vi "Sys config window-Get set control values_retd.vi"(8 "error in (no error)":errorcluster, 11 "Function":T28) -> (0 "error out":errorcluster, 2 "output cluster":T1={"Triggers output setup"=[], "General trigger settings"={"Trigger 1 function"=enum."Encoder trigger", "Triggers loop clock (MHz)"=80.0}, "AOL Properties"={"AOD 1 thickness (mm)"=118.0, "AOD 2 thickness (mm)"=115.0, "AOD 3 thickness (mm)"=110.0, "AOD 4 thickness (mm)"=135.0, "AOD 5 thickness (mm)"=135.0, "AOD 6 thickness (mm)"=135.0, "AOD 1-2 separation (mm)"=15.0, "AOD 2-3 separation (mm)"=15.0, "AOD 3-4 separation (mm)"=15.0, "AOD 4-5 separation (mm)"=15.0, "AOD 5-6 separation (mm)"=15.0, "AOD 1 X Offset"=15.0, "AOD 2 X Offset"=1.0, "AOD 3 X Offset"=1.0, "AOD 4 X Offset"=1.0, "AOD 1 Y Offset"=1.0, "AOD 2 Y Offset"=1.0, "AOD 3 Y Offset"=1.0, "AOD 4 Y Offset"=1.0, "AOD 1 X Direction"=0.0, "AOD 2 X Direction"=0.0, "AOD 3 X Direction"=0.0, "AOD 4 X Direction"=0.0, "AOD 1 Y Direction"=1.0, "AOD 2 Y Direction"=20000.0, "AOD 3 Y Direction"=20000.0, "AOD 4 Y Direction"=0.0046, "AOD 1 Centre (mm)"=15.0, "AOD 2 Centre (mm)"=50.0, "AOD 3 Centre (mm)"=50.0, "AOD 4 Centre (mm)"=50.0, "Timing Offset AOD 1"=0.0, "Timing Offset AOD 2"=0.0, "Timing Offset AOD 3"=0.0, "Timing Offset AOD 4"=0.0, "AOD Optical offset 1"=0.0, "AOD Optical offset 2"=0.0, "AOL aperture (mm)"=15.0, "AOL centre wavelength (nm)"=1.0, "AOL centre frequency (MHz)"=1.0, "Diffraction mode"=1.0, "Crystal length (mm)"=0.0, "Acoustic velocity (m/s)"=1.0, "Pair deflection ratio"=1.0, "AOD fill time (us)"=1.0, "AOD Ord. Refractive index"=2.22, "AOD ExtraOrd. Refractive index"=2.22}, "Calibration settings"={"Pockels cal.Zoom"=0, "Pockels cal.Dwell time (µs)"=0.0}, "Hardware Configuration"={"Microscope ID"="003", "Microscope Type"="AOLM", "Revision Number"="1.0.0.0", "Advanced Imaging"=FALSE, "Max Allowed Trial Length"=60.0, "Initial Scan Resolution"=512.0, "Initial Acceptance Angle"=5.0, "Dev. PC"=FALSE, "Swap XY on stage"=FALSE, "No of AOD"=0, "MC Supported"=FALSE, "Axial MC"=FALSE, "Computer MAC address"="", "Externalise Triggers"=FALSE, "Trigger HW config"={"Available Device List"=0, "Device Address"=""}, "DAQmx Chan"={"Pockels AO"="", "Hard shutter AO"="", "PMT AOs"="", "Galvo AOs"="", "Power meter AI"=""}, "XY stage available"=FALSE, "XY Stage"={"COM port"="", "XY stage available"=FALSE, "Baudrate"=0, "Type"=""}, "Z stage available"=FALSE, "Z Stage config cluster"={"COM port"="COM7", "Baudrate"=0, "Type"=""}, "Encoder available"=FALSE, "Encoder"={"IP address"="224.0.1.103", "Port"=7000, "Wheel radius (cm)"=16.0, "Encoder Trigger"=""}, "VidRec available"=FALSE, "Cam VidRec"={"DO flag-Video record"="", "DO flag-Trial start"=""}, "Laser Power Control HW config"={"Laser Power Control"="", "Laser Power Modulation Control"=enum."NI"}, "Laser 1 available"=FALSE, "Laser 1 config cluster"={"COM port"="COM7", "Baud Rate"=0, "Type"=""}, "Prechirper 1 available"=FALSE, "Prechirper 1 config cluster"={"Type"="", "Baud Rate"=0, "COM port"="COM7"}, "Control system.FPGA available?"=FALSE, "Control Sys. HW config"={"Control system.FPGA Type"=enum."Virtex 5", "Control system.Network adapter name"="", "Control system.MAC address"="", "Control system.Ethernet Port"=0, "Control system.Ethernet Port Opened"=FALSE}, "DAQ FPGA HW Config"={"Target"="RIO0", "input card type"=enum."AC Card"}}, "System Config"={"Laser wavelength (nm)"=920.0, "DAQ FPGA System"={"Clock Freq (MHz) "=200.0, "Samples Wait after Trigger"=5080, "AOD fill"=4900, "StartupDelay"=0, "Slip Cycle (clock cycles)"=600000, "Add Cycle"=TRUE}, "Control system"={"AOD 1 Amplitude"=0, "AOD 2 Amplitude"=0, "AOD 3 Amplitude"=0, "AOD 4 Amplitude"=0, "AOD 5 Amplitude"=0, "AOD 6 Amplitude"=0, "T0 (ns)"=0.0, "Ta (ns)"=0.0, "Data Time Interval (ns)"=0.0, "Ctrl FPGA Clock (MHz)"=240.0}}, "Calibration config."={"Current Objective"="", "Objective Settings"=[], "PreChirper Values Preset ?"=FALSE, "PreChirper Settings"=[], "PreChirper Constants"={"a 1"=0, "b 1"=0, "c 1"=0, "a 2"=0, "b 2"=0, "c 2"=0, "lmin"=0, "lmax"=0}}} {"System Config"."Control system"."Ctrl FPGA Clock (MHz)" min=80.0 max=500.0 step=1.0; "System Config"."Control system"."Data Time Interval (ns)" min=0.0 max=2048.0 step=1.0; "System Config"."Control system"."Ta (ns)" min=0.0 max=2048.0 step=1.0; "System Config"."Control system"."T0 (ns)" min=0.0 max=2048.0 step=1.0; "System Config"."Control system"."AOD 6 Amplitude" min=0 max=2048 step=1; "System Config"."Control system"."AOD 5 Amplitude" min=0 max=2048 step=1; "System Config"."Control system"."AOD 4 Amplitude" min=0 max=2048 step=1; "System Config"."Control system"."AOD 3 Amplitude" min=0 max=2048 step=1; "System Config"."Control system"."AOD 2 Amplitude" min=0 max=2048 step=1; "System Config"."Control system"."AOD 1 Amplitude" min=0 max=2048 step=1; "System Config"."Laser wavelength (nm)" min=800.0 max=1080.0 step=1.0; "Hardware Configuration"."Encoder"."Wheel radius (cm)" format="%#_13g"; "General trigger settings"."Triggers loop clock (MHz)" format="%#_13g"; "Triggers output setup"."Pulse width (us)" min=10 max=5000 step=1 format="%.0fµs"})   [LabVIEW 2020]
uses:
  Typedefs/HW config states enum.ctl
  Globals/Sys Config window globals.vi
  Configuration code/Calibration/Globals/gl_Calibration globals.vi
  Configuration code/Typedefs/Pockels Calibration settings cluster.ctl
  Global Variables/General Globals.vi
  Peripherals Control/Triggers/Typedefs/Trigger setup element cluster.ctl
  Peripherals Control/Triggers/Typedefs/Triggers output setup.ctl
  Typedefs/Trigger 1 selector enum.ctl
  Peripherals Control/Triggers/Typedefs/General trigger settings cluster.ctl
  Typedefs/XY Stage config cluster.ctl
  Typedefs/Cam VidRec HW config setup cluster.ctl
  Typedefs/Control Sys HW config cluster.ctl
  <vilib>/userDefined/High Color/nirio_resource_hc.ctl
  Typedefs/FPGA input type AC-DC.ctl
  Typedefs/DAQmx physical channels cluster.ctl
  Typedefs/Encoder config cluster.ctl
  Typedefs/Z Stage config cluster.ctl
  Typedefs/Triggers HW config.ctl
  Typedefs/Laser 1 config cluster.ctl
  Typedefs/PreChirper 1 config cluster.ctl
  Typedefs/Laser Power Control HW config.ctl
  Typedefs/Hardware Configuration settings.ctl
  RIG-SPECIFIC FILES/FPGA Refs/FPGA Ref.ctl
  Typedefs/DAQ FPGA system config.ctl
  Typedefs/CTRL system config.ctl
  Typedefs/System Configuration.ctl
  Configuration code/Typedefs/Initial config.ctl
  Typedefs/PreChirper constants.ctl
  Typedefs/Prechirper Cal Config.ctl
  Typedefs/Objective Config.ctl
  Typedefs/Calibration config.ctl
  Typedefs/AOD Settings-distilled.ctl
  Typedefs/General Setup.ctl
  Typedefs/PMT Voltage Range.ctl
  Typedefs/DAQ FPGA HW config cluster.ctl
  Visualisation/Functional Imaging Viewer/Typedefs/Get-Set-Clear Control.ctl
  Typedefs/AOL Properties Cluster.ctl
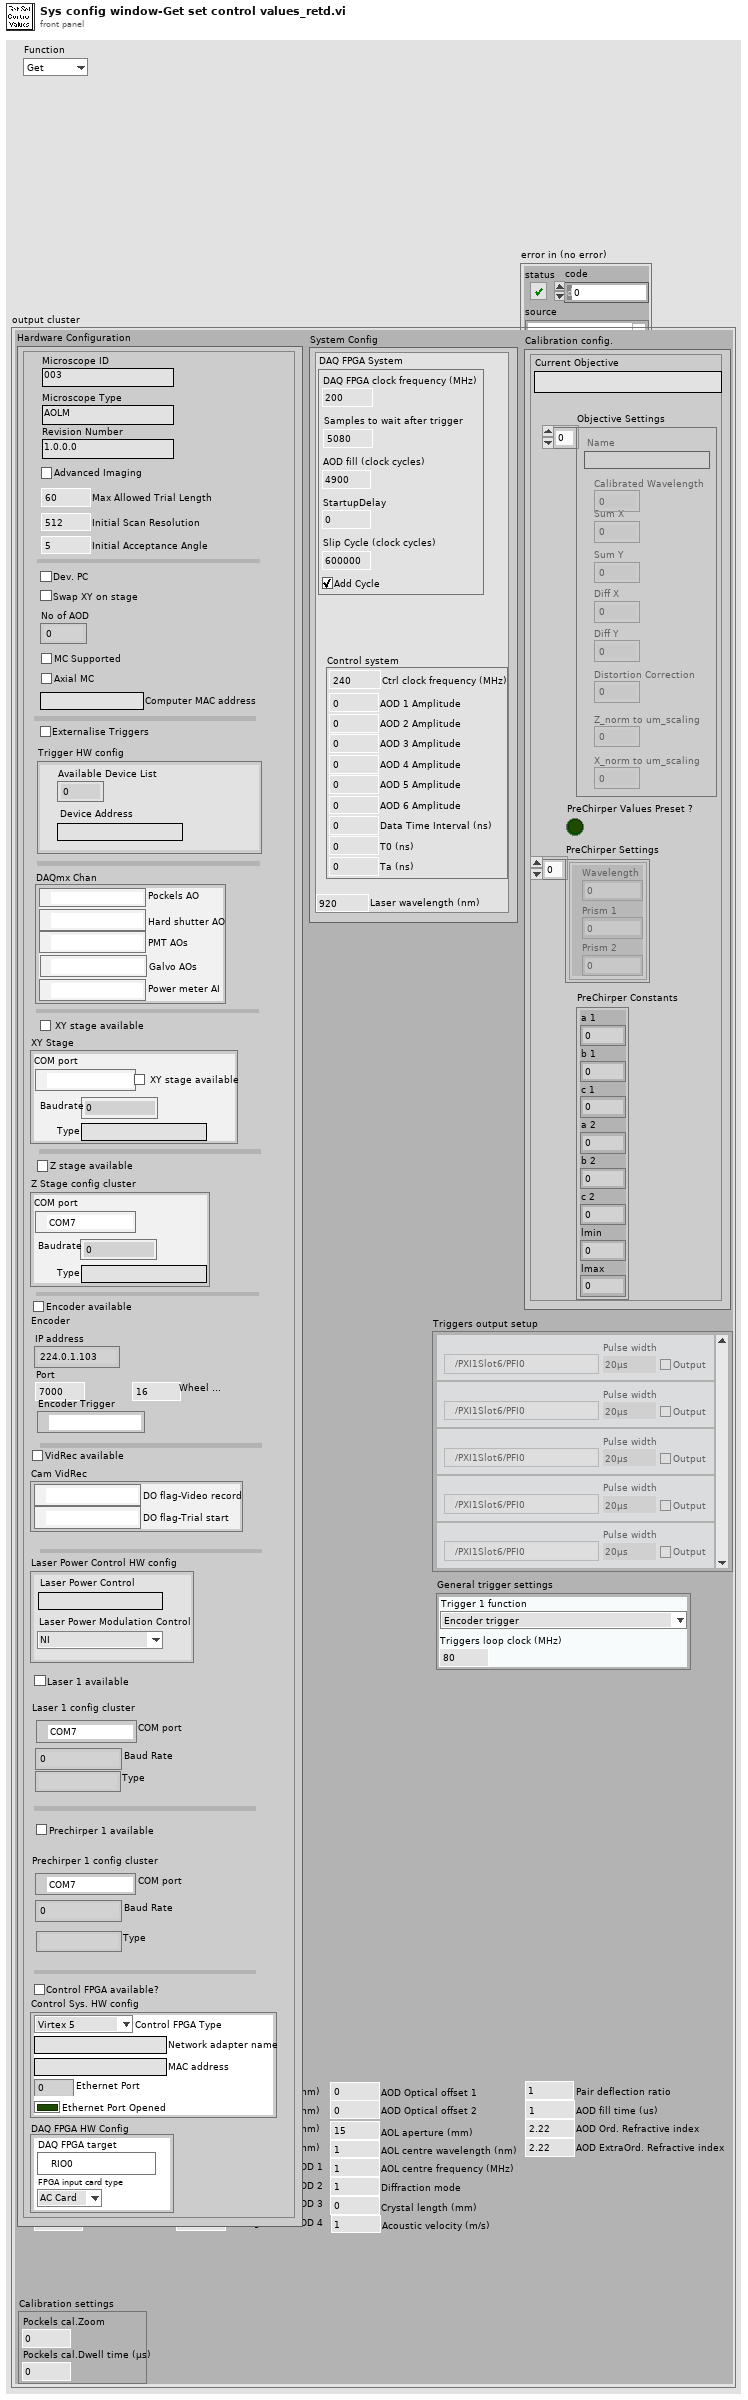
[diagram p1: front panel]
types:
  T1 = typedef "Initial config.ctl" = cluster{"Triggers output setup":T2, "General trigger settings":T4, "AOL Properties":T6, "Calibration settings":T7, "Hardware Configuration":T8, "System Config":T21, "Calibration config.":T24}
  T2 = typedef "Triggers output setup.ctl" = T3[]
  T3 = typedef "Trigger setup element cluster.ctl" = cluster{"Name":string, "Output?":bool, "Output terminal":tag, "PXI backplane line":tag, "Pulse width (us)":u16}
  T4 = typedef "General trigger settings cluster.ctl" = cluster{"Trigger 1 function":T5, "Triggers loop clock (MHz)":dbl}
  T5 = typedef "Trigger 1 selector enum.ctl" = enum16{"Encoder trigger", "Line trigger", "Control system's ref frame acknowledgement"}
  T6 = typedef "AOL Properties Cluster.ctl" = cluster{"AOD 1 thickness (mm)":dbl, "AOD 2 thickness (mm)":dbl, "AOD 3 thickness (mm)":dbl, "AOD 4 thickness (mm)":dbl, "AOD 5 thickness (mm)":dbl, "AOD 6 thickness (mm)":dbl, "AOD 1-2 separation (mm)":dbl, "AOD 2-3 separation (mm)":dbl, "AOD 3-4 separation (mm)":dbl, "AOD 4-5 separation (mm)":dbl, "AOD 5-6 separation (mm)":dbl, "AOD 1 X Offset":dbl, "AOD 2 X Offset":dbl, "AOD 3 X Offset":dbl, "AOD 4 X Offset":dbl, "AOD 1 Y Offset":dbl, "AOD 2 Y Offset":dbl, "AOD 3 Y Offset":dbl, "AOD 4 Y Offset":dbl, "AOD 1 X Direction":dbl, "AOD 2 X Direction":dbl, "AOD 3 X Direction":dbl, "AOD 4 X Direction":dbl, "AOD 1 Y Direction":dbl, "AOD 2 Y Direction":dbl, "AOD 3 Y Direction":dbl, "AOD 4 Y Direction":dbl, "AOD 1 Centre (mm)":dbl, "AOD 2 Centre (mm)":dbl, "AOD 3 Centre (mm)":dbl, "AOD 4 Centre (mm)":dbl, "Timing Offset AOD 1":dbl, "Timing Offset AOD 2":dbl, "Timing Offset AOD 3":dbl, "Timing Offset AOD 4":dbl, "AOD Optical offset 1":dbl, "AOD Optical offset 2":dbl, "AOL aperture (mm)":dbl, "AOL centre wavelength (nm)":dbl, "AOL centre frequency (MHz)":dbl, "Diffraction mode":dbl, "Crystal length (mm)":dbl, "Acoustic velocity (m/s)":dbl, "Pair deflection ratio":dbl, "AOD fill time (us)":dbl, "AOD Ord. Refractive index":dbl, "AOD ExtraOrd. Refractive index":dbl}
  T7 = typedef "Pockels Calibration settings cluster.ctl" = cluster{"Pockels cal.Zoom":u8, "Pockels cal.Dwell time (µs)":dbl}
  T8 = typedef "Hardware Configuration settings.ctl" = cluster{"Microscope ID":string, "Microscope Type":string, "Revision Number":string, "Advanced Imaging":bool, "Max Allowed Trial Length":dbl, "Initial Scan Resolution":dbl, "Initial Acceptance Angle":dbl, "Dev. PC":bool, "Swap XY on stage":bool, "No of AOD":u8, "MC Supported":bool, "Axial MC":bool, "Computer MAC address":string, "Externalise Triggers":bool, "Trigger HW config":T9, "DAQmx Chan":T10, "XY stage available":bool, "XY Stage":T11, "Z stage available":bool, "Z Stage config cluster":T12, "Encoder available":bool, "Encoder":T13, "VidRec available":bool, "Cam VidRec":T14, "Laser Power Control HW config":T15, "Laser 1 available":bool, "Laser 1 config cluster":T16, "Prechirper 1 available":bool, "Prechirper 1 config cluster":T17, "Control system.FPGA available?":bool, "Control Sys. HW config":T18, "DAQ FPGA HW Config":cluster{"Target":T19, "input card type":T20}}
  T9 = typedef "Triggers HW config.ctl" = cluster{"Available Device List":i32, "Device Address":string}
  T10 = typedef "DAQmx physical channels cluster.ctl" = cluster{"Pockels AO":tag, "Hard shutter AO":tag, "PMT AOs":tag, "Galvo AOs":tag, "Power meter AI":tag}
  T11 = typedef "XY Stage config cluster.ctl" = cluster{"COM port":refnum<visa-resource-name>, "XY stage available":bool, "Baudrate":i32, "Type":string}
  T12 = typedef "Z Stage config cluster.ctl" = cluster{"COM port":refnum<visa-resource-name>, "Baudrate":i32, "Type":string}
  T13 = typedef "Encoder config cluster.ctl" = cluster{"IP address":string, "Port":u16, "Wheel radius (cm)":dbl, "Encoder Trigger":tag}
  T14 = typedef "Cam VidRec HW config setup cluster.ctl" = cluster{"DO flag-Video record":tag, "DO flag-Trial start":tag}
  T15 = typedef "Laser Power Control HW config.ctl" = cluster{"Laser Power Control":string, "Laser Power Modulation Control":enum16{"NI", "FPGA"}}
  T16 = typedef "Laser 1 config cluster.ctl" = cluster{"COM port":refnum<visa-resource-name>, "Baud Rate":i32, "Type":string}
  T17 = typedef "PreChirper 1 config cluster.ctl" = cluster{"Type":string, "Baud Rate":i32, "COM port":refnum<visa-resource-name>}
  T18 = typedef "Control Sys HW config cluster.ctl" = cluster{"Control system.FPGA Type":enum16{"Virtex 5", "Virtex 7"}, "Control system.Network adapter name":string, "Control system.MAC address":string, "Control system.Ethernet Port":u32, "Control system.Ethernet Port Opened":bool}
  T19 = typedef "nirio_resource_hc.ctl" = tag
  T20 = typedef "FPGA input type AC-DC.ctl" = enum16{"AC Card", "DC Card"}
  T21 = typedef "System Configuration.ctl" = cluster{"Laser wavelength (nm)":dbl, "DAQ FPGA System":T22, "Control system":T23}
  T22 = typedef "DAQ FPGA system config.ctl" = cluster{"Clock Freq (MHz) ":dbl, "Samples Wait after Trigger":u16, "AOD fill":u16, "StartupDelay":i32, "Slip Cycle (clock cycles)":u32, "Add Cycle":bool}
  T23 = typedef "CTRL system config.ctl" = cluster{"AOD 1 Amplitude":i16, "AOD 2 Amplitude":i16, "AOD 3 Amplitude":i16, "AOD 4 Amplitude":i16, "AOD 5 Amplitude":i16, "AOD 6 Amplitude":i16, "T0 (ns)":dbl, "Ta (ns)":dbl, "Data Time Interval (ns)":dbl, "Ctrl FPGA Clock (MHz)":dbl}
  T24 = typedef "Calibration config.ctl" = cluster{"Current Objective":string, "Objective Settings":T25[], "PreChirper Values Preset ?":bool, "PreChirper Settings":T26[], "PreChirper Constants":T27}
  T25 = typedef "Objective Config.ctl" = cluster{"Name":string, "Sum X":dbl, "Sum Y":dbl, "Diff X":dbl, "Diff Y":dbl, "Distortion Correction":dbl, "Z_norm to um_scaling":dbl, "X_norm to um_scaling":dbl, "Calibrated Wavelength":dbl}
  T26 = typedef "Prechirper Cal Config.ctl" = cluster{"Wavelength":i32, "Prism 1":i32, "Prism 2":i32}
  T27 = typedef "PreChirper constants.ctl" = cluster{"a 1":i32, "b 1":i32, "c 1":i32, "a 2":i32, "b 2":i32, "c 2":i32, "lmin":i32, "lmax":i32}
  T28 = typedef "Get-Set-Clear Control.ctl" = enum16{"Get", "Set", "Clear"}
  T29 = enum16{"Initialise", "Load from file", "Save to file", "Read", "Write"}
  T30 = typedef "Initial config.ctl" = cluster{"Triggers output setup":T2, "General trigger settings":T4, "Calibration settings":T7, "Hardware Configuration":T31, "System Config":T21, "Calibration config.":T24, "General Setup":T36, "AOD Settings - distilled":T37}
  T31 = typedef "Hardware Configuration settings.ctl" = cluster{"Dev. PC":bool, "Swap XY on stage":bool, "No of AOD":u8, "MC Supported":bool, "Axial MC":bool, "Computer MAC address":string, "Externalise Triggers":bool, "Trigger HW config":T9, "DAQmx Chan":T10, "XY stage available":bool, "XY Stage":T32, "Z stage available":bool, "Z Stage config cluster":T12, "Encoder available":bool, "Encoder":T13, "VidRec available":bool, "Cam VidRec":T14, "Laser Power Control HW config":T15, "Laser 1 available":bool, "Laser 1 config cluster":T16, "Prechirper 1 available":bool, "Prechirper 1 config cluster":T17, "Control system.FPGA available?":bool, "Control Sys. HW config":T18, "DAQ FPGA HW Config":T33, "PMT Voltage Range":T35}
  T32 = typedef "XY Stage config cluster.ctl" = cluster{"COM port":refnum<visa-resource-name>, "Baudrate":i32, "Type":string}
  T33 = typedef "DAQ FPGA HW config cluster.ctl" = cluster{"FGPA Ref":T34, "Target":T19, "input card type":T20}
  T34 = typedef "FPGA Ref.ctl" = refnum<k20>
  T35 = typedef "PMT Voltage Range.ctl" = cluster{"PMT Voltage Lower Limit":dbl, "PMT Voltage Upper Limit":dbl}
  T36 = typedef "General Setup.ctl" = cluster{"Microscope ID":string, "Microscope Type":string, "Revision Number":string, "Advanced Imaging":bool, "Error Logging":bool, "Performance Monitoring":bool, "Max Allowed Trial Length":dbl, "Initial Scan Resolution":dbl, "Initial Acceptance Angle":dbl, "Initial Laser Wavelength":dbl, "Initial Dwell Time":dbl}
  T37 = typedef "AOD Settings-distilled.ctl" = cluster{"AOD 1 thickness (mm)":dbl, "AOD 2 thickness (mm)":dbl, "AOD 3 thickness (mm)":dbl, "AOD 4 thickness (mm)":dbl, "AOD 1-2 separation (mm)":dbl, "AOD 2-3 separation (mm)":dbl, "AOD 3-4 separation (mm)":dbl, "AOD 1 Centre (mm)":dbl, "AOD 2 Centre (mm)":dbl, "AOD 3 Centre (mm)":dbl, "AOD 4 Centre (mm)":dbl, "AOD 1 X Offset":dbl, "AOD 2 X Offset":dbl, "AOD 3 X Offset":dbl, "AOD 4 X Offset":dbl, "AOD 1 Y Offset":dbl, "AOD 2 Y Offset":dbl, "AOD 3 Y Offset":dbl, "AOD 4 Y Offset":dbl, "Timing Offset AOD 1":dbl, "Timing Offset AOD 2":dbl, "Timing Offset AOD 3":dbl, "Timing Offset AOD 4":dbl, "AOL centre wavelength (nm)":dbl, "AOL centre frequency (MHz)":dbl, "Pair deflection ratio":dbl, "AOL aperture (mm)":dbl, "AOD fill time (us)":dbl, "Diffraction mode":dbl, "Crystal length (mm)":dbl, "Acoustic velocity (m/s)":dbl, "AOD Ord. Refractive index":dbl}
  T38 = typedef "HW config states enum.ctl" = enum16{"Load from file", "Save to file", "Save backup", "Write all", "Read all", "Write XY stage settings", "Write DAQ FPGA settings", "Write Control FPGA settings", "Write Phys Channels", "Write System Config", "Write HW Config", "Save System Config", "Save HW Config", "Clear", "Compare from file"}
  T39 = typedef "HW config window refs cluster.ctl" = cluster{"VI's reference":refnum<vi>, "menu reference":refnum<k9>, "Pane":refnum<vi>, "Config Tab Control":refnum<vi>, "Triggers sub-tab control":refnum<vi>, "Microscope ID":refnum<vi>, "Microscope Type":refnum<vi>, "Revision Number":refnum<vi>, "Advanced Imaging":refnum<vi>, "Max Allowed Trial Length":refnum<vi>, "Initial Scan Resolution":refnum<vi>, "Initial Acceptance Angle":refnum<vi>, "Initial Laser Wavelength [nm] ":refnum<vi>, "Initial Dwell Time [us]":refnum<vi>, "Error Logging":refnum<vi>, "Performance Monitoring":refnum<vi>, "Ctrl FPGA available":refnum<vi>, "Control HW config":refnum<vi>, "Control System Config":refnum<vi>, "General trigger settings":refnum<vi>, "Trigger HW config":refnum<vi>, "Externalise Triggers":refnum<vi>, "[Triggers output setup]":refnum<vi>, "DAQ FPGA HW Config":refnum<vi>, "DAQ FPGA System Config":refnum<vi>, "Pockels AO":refnum<vi>, "Hard shutter AO":refnum<vi>, "PMT AOs":refnum<vi>, "Galvo AO":refnum<vi>, "Power meter AI":refnum<vi>, "XY stage available":refnum<vi>, "XY Stage config cluster":refnum<vi>, "Z stage available":refnum<vi>, "Z Stage config cluster":refnum<vi>, "Encoder available":refnum<vi>, "Encoder":refnum<vi>, "Encoder IP address":refnum<vi>, "Encoder port":refnum<vi>, "Wheel radius (cm)":refnum<vi>, "Demo mode":refnum<vi>, "Swap XY on stage":refnum<vi>, "Number of AODs":refnum<vi>, "Axial MC Supported":refnum<vi>, "MC Supported":refnum<vi>, "Computer MAC add.":refnum<vi>, "Cam VidRec available":refnum<vi>, "Cam VidRec":refnum<vi>, "DO flag-Video record":refnum<vi>, "DO flag-Trial start":refnum<vi>, "AOD Settings (distilled)":refnum<vi>, "Pockels cal.Dwell time (µs)":refnum<vi>, "Pockels cal.Zoom":refnum<vi>, "Current Objective":refnum<vi>, "[Obj. Calib. Settings]":refnum<vi>, "Laser Wavelength":refnum<vi>, "Laser Power Control \nHW config":refnum<vi>, "Laser 1 available":refnum<vi>, "Laser 1 config":refnum<vi>, "Prechirper 1 available":refnum<vi>, "Prechirper 1 config":refnum<vi>, "PreChirp Preset Values":refnum<vi>, "[PreChirper Preset \nCalibration Values]":refnum<vi>, "Prechirper Constants":refnum<vi>}
  T40 = typedef "DAQ FPGA config cluster.ctl" = cluster{"Target":T19, "input card type":T20, "Ref":T34, "Clock Freq (MHz) ":dbl, "Samples Wait after Trigger":u16, "AOD fill":u16, "StartupDelay":i32, "Slip Cycle (clock cycles)":u32, "Add Cycle":bool}
  T41 = typedef "CTRL system config cluster.ctl" = cluster{"Ctrl FPGA available":bool, "Control system.FPGA Type":string, "Control system.Network adapter name":string, "Control system.MAC address":string, "Control system.Ethernet Port":i16, "Ethernet opened":bool, "Ctrl FPGA Clock (MHz)":dbl, "AOD 1 Amplitude":i16, "AOD 2 Amplitude":i16, "AOD 3 Amplitude":i16, "AOD 4 Amplitude":i16, "AOD 5 Amplitude":i16, "AOD 6 Amplitude":i16, "Data Time Interval (ns)":dbl, "T0 (ns)":dbl, "Ta (ns)":dbl, "Ethernet Port":u32}
  T42 = typedef "AOL Properties Cluster.ctl" = cluster{"AOD 1 thickness (mm)":dbl, "AOD 2 thickness (mm)":dbl, "AOD 3 thickness (mm)":dbl, "AOD 4 thickness (mm)":dbl, "AOD 5 thickness (mm)":dbl, "AOD 6 thickness (mm)":dbl, "AOD 1-2 separation (mm)":dbl, "AOD 2-3 separation (mm)":dbl, "AOD 3-4 separation (mm)":dbl, "AOD 4-5 separation (mm)":dbl, "AOD 5-6 separation (mm)":dbl, "AOD 1 Centre (mm)":dbl, "AOD 2 Centre (mm)":dbl, "AOD 3 Centre (mm)":dbl, "AOD 4 Centre (mm)":dbl, "AOD 1 X Offset":dbl, "AOD 2 X Offset":dbl, "AOD 3 X Offset":dbl, "AOD 4 X Offset":dbl, "AOD 1 Y Offset":dbl, "AOD 2 Y Offset":dbl, "AOD 3 Y Offset":dbl, "AOD 4 Y Offset":dbl, "Diffraction mode":dbl, "Crystal length (mm)":dbl, "Acoustic velocity (m/s)":dbl, "AOD fill time (us)":dbl, "AOD Ord. Refractive index":dbl, "AOL aperture (mm)":dbl, "AOL centre wavelength (nm)":dbl, "AOL centre frequency (MHz)":dbl, "Pair deflection ratio":dbl, "Sum X":dbl, "Sum Y":dbl, "Diff X":dbl, "Diff Y":dbl, "Timing Offset AOD 1":dbl, "Timing Offset AOD 2":dbl, "Timing Offset AOD 3":dbl, "Timing Offset AOD 4":dbl, "Distortion Correction":dbl, "Z_norm to um_scaling":dbl, "X_norm to um_scaling":dbl}
  T43 = typedef "CTRL system config cluster.ctl" = cluster{"Contrl Sys Available Ind":bool, "Control system.FPGA Type":enum16{"Virtex 5", "Virtex 7"}, "Control system.Network adapter name":string, "Control system.MAC address":string, "Control system.Ethernet Port":i16, "Ethernet opened":bool, "Ctrl FPGA Clock (MHz)":dbl, "AOD 1 Amplitude":i16, "AOD 2 Amplitude":i16, "AOD 3 Amplitude":i16, "AOD 4 Amplitude":i16, "AOD 5 Amplitude":i16, "AOD 6 Amplitude":i16, "Data Time Interval (ns)":dbl, "T0 (ns)":dbl, "Ta (ns)":dbl}
  T44 = typedef "CTRL system config cluster ref.ctl" = refnum<vi>
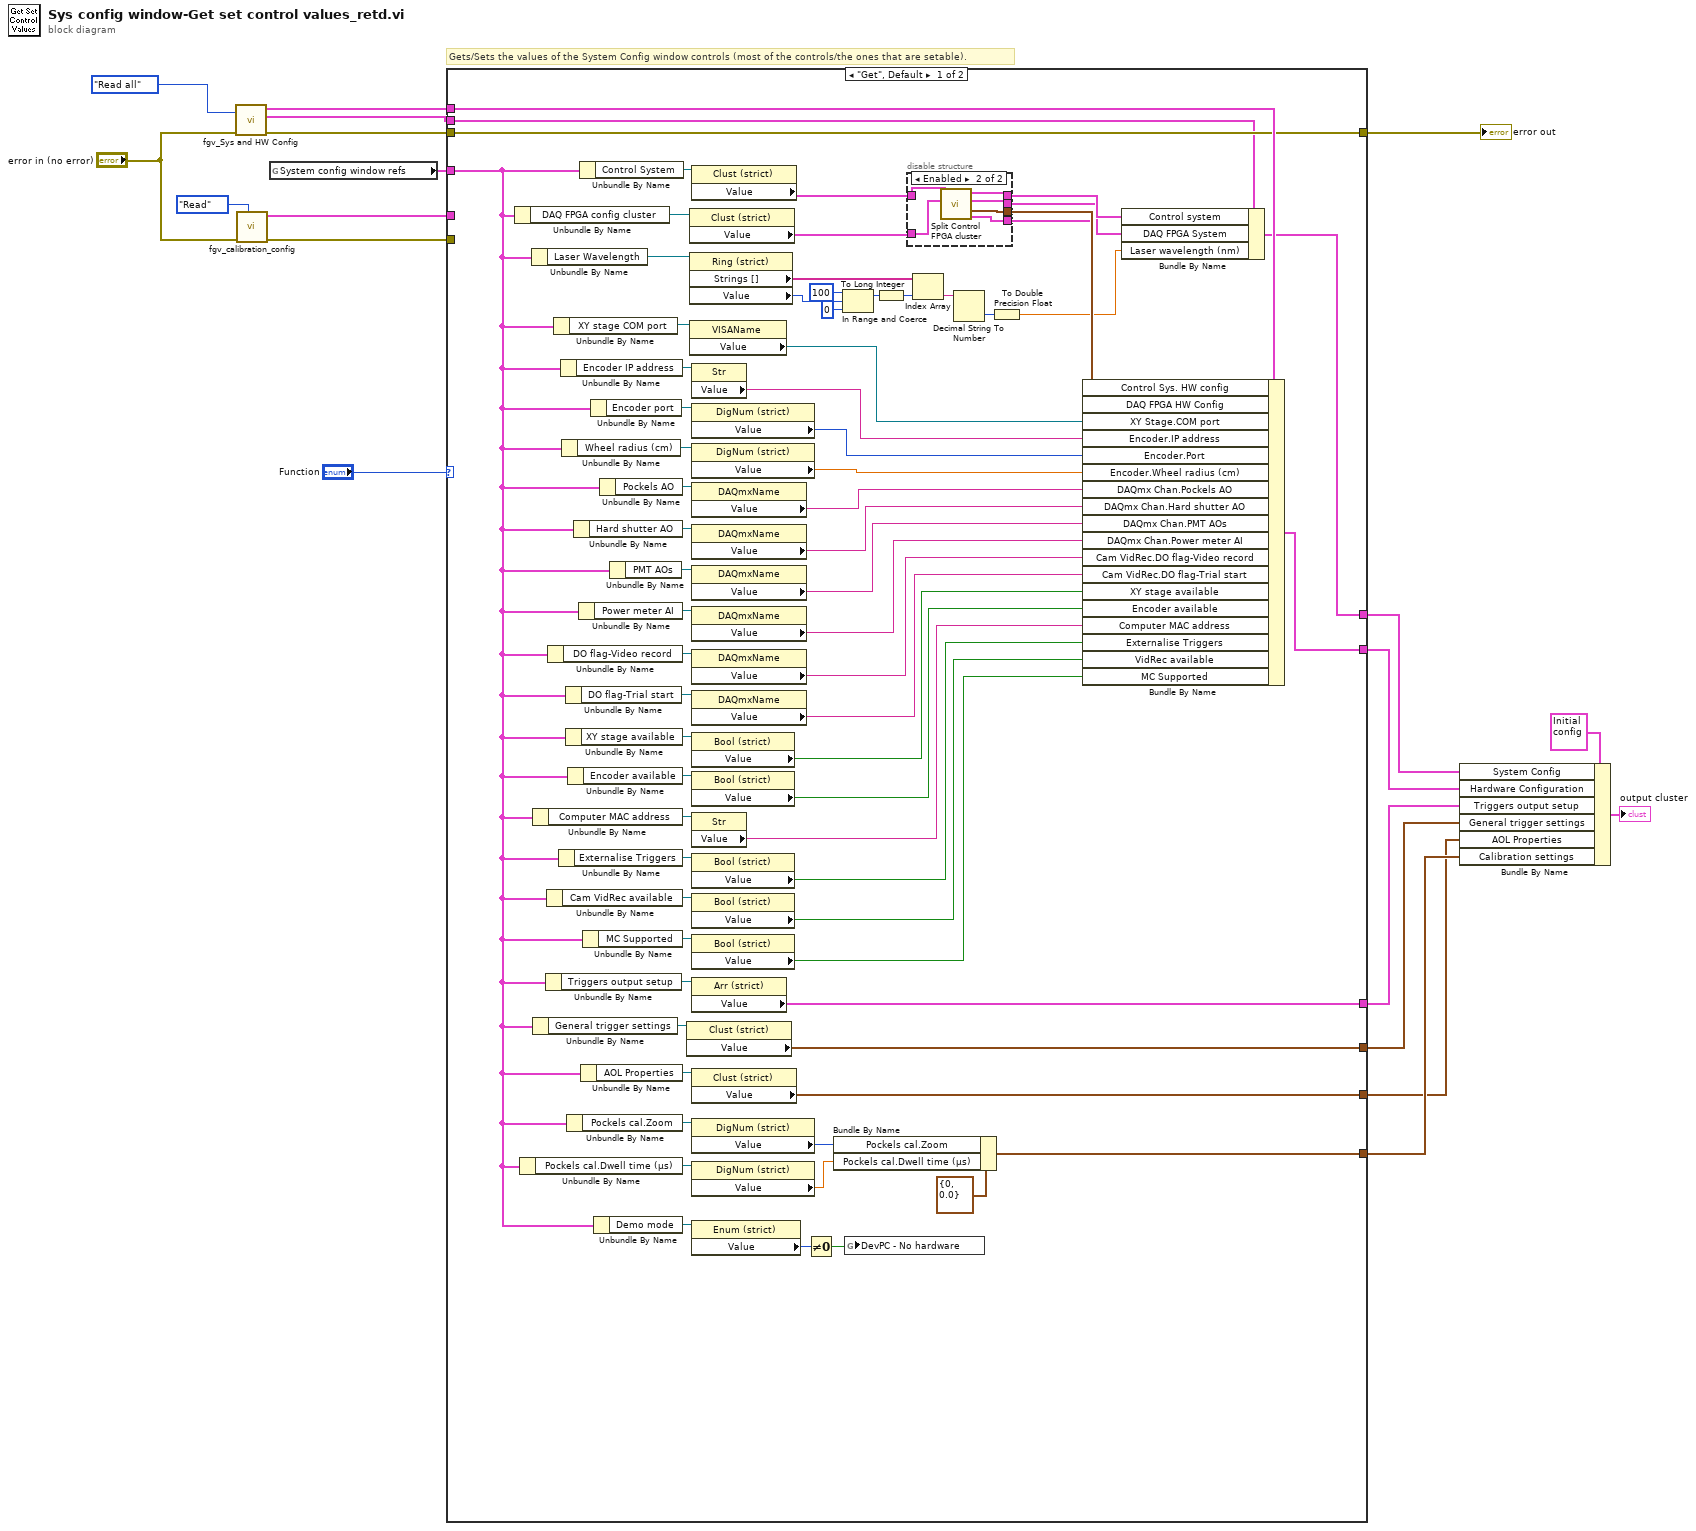
[diagram p0: block diagram]
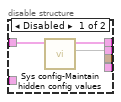
[diagram p2: hidden frame]
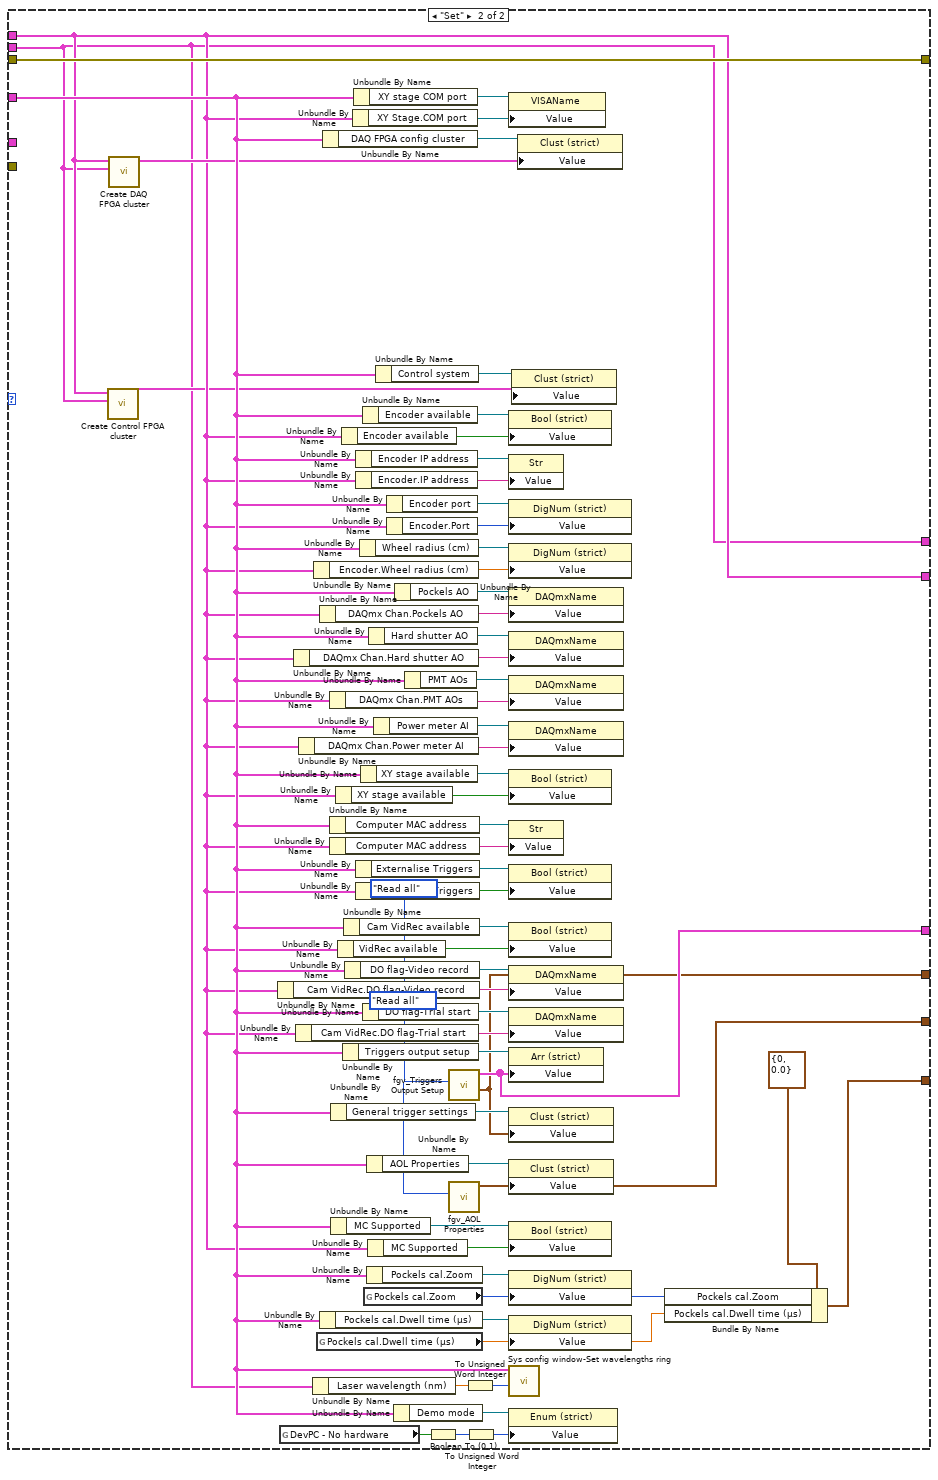
[diagram p3: hidden frame]
diagram:
  # "Gets/Sets the values of the System Config window controls (most of the controls/the ones that are setable)."
  n1 = call "fgv_Sys and HW Config.vi"("Function"=HW_config_states_enum."Read all", "error in (no error)"="error in (no error)") -> ("error out"=w14:errorcluster, "System Config OUT"=w10:T21, "Hardware Configuration OUT"=w15:T31)  [unwired: 7 in]
  n2 = call "fgv_calibration_config.vi"("Cal config ops"=T29."Read", "error in (no error)"="error in (no error)") -> ("error out"=w1:errorcluster, "Config cluster OUT"=w2:T24)  [unwired: 7 in, 1 out]
  n3 = global read "Sys Config window globals.vi" "System config window refs"() -> (w19:T39)
  n4 = case shown="\"Get\", Default" "Function" {
    tunnel: w19 -> [w31 w105]
    tunnel: [w74 w102] -> w7
    tunnel: [w56 w123] -> w17
    tunnel: [w62 w125] -> w16
    tunnel: [w60 w129] -> w12
    tunnel: w15 -> [w57 w102]
    tunnel: w14 -> [w56 w123]
    tunnel: [w51 w117] -> w13
    tunnel: [w30 w104] -> w11
    tunnel: w10 -> [w29 w100]
    tunnel: [w27 w100] -> w6
    tunnel: w2 -> [_ _]
    tunnel: w1 -> [_ _]
    frame "Get", Default {
      n5 = Unbundle By Name(w31) -> ("DAQ FPGA config cluster"=w76:refnum<vi>)
      n6 = Unbundle By Name(w31) -> ("Pockels cal.Dwell time (µs)"=w55:refnum<vi>)
      n7 = Unbundle By Name(w31) -> ("Laser Wavelength"=w50:refnum<vi>)
      n8 = Unbundle By Name(w31) -> ("Computer MAC address"=w69:refnum<vi>)
      n9 = Unbundle By Name(w31) -> ("General trigger settings"=w32:refnum<vi>)
      n10 = Unbundle By Name(w31) -> ("Triggers output setup"=w63:refnum<vi>)
      n11 = Unbundle By Name(w31) -> ("Cam VidRec available"=w65:refnum<vi>)
      n12 = Unbundle By Name(w31) -> ("DO flag-Video record"=w79:refnum<vi>)
      n13 = Unbundle By Name(w31) -> ("XY stage COM port"=w75:refnum<vi>)
      n14 = Unbundle By Name(w31) -> ("Externalise Triggers"=w67:refnum<vi>)
      n15 = Unbundle By Name(w31) -> ("Encoder IP address"=w78:refnum<vi>)
      n16 = Unbundle By Name(w31) -> ("Wheel radius (cm)"=w37:refnum<vi>)
      n17 = Unbundle By Name(w31) -> ("DO flag-Trial start"=w84:refnum<vi>)
      n18 = Unbundle By Name(w31) -> ("XY stage available"=w73:refnum<vi>)
      n19 = Unbundle By Name(w31) -> ("Pockels cal.Zoom"=w54:refnum<vi>)
      n20 = Unbundle By Name(w31) -> ("Encoder available"=w72:refnum<vi>)
      n21 = Unbundle By Name(w31) -> ("Hard shutter AO"=w81:refnum<vi>)
      n22 = Unbundle By Name(w31) -> ("Power meter AI"=w39:refnum<vi>)
      n23 = Unbundle By Name(w31) -> ("Control System"=w77:refnum<vi>)
      n24 = Unbundle By Name(w31) -> ("AOL Properties"=w61:refnum<vi>)
      n25 = Unbundle By Name(w31) -> ("MC Supported"=w59:refnum<vi>)
      n26 = Unbundle By Name(w31) -> ("Encoder port"=w83:refnum<vi>)
      n27 = Unbundle By Name(w31) -> ("Demo mode"=w35:refnum<vi>)
      n28 = Unbundle By Name(w31) -> ("Pockels AO"=w82:refnum<vi>)
      n29 = Unbundle By Name(w31) -> ("PMT AOs"=w80:refnum<vi>)
      n30 = property class="Clust (strict)"(reference=w32) -> ("Value"=w30:T4)  [unwired: 1 in, 2 out]
      n31 = property class="Clust (strict)"(reference=w76) -> ("Value"=w24:T40)  [unwired: 1 in, 2 out]
      n32 = property on="Property Node" class="Ring (strict)"(reference=w50) -> ("Strings []"=w49:string[], "Value"=w46:u16)  [unwired: 1 in, 2 out]
      n33 = property class="VISAName"(reference=w75) -> ("Value"=w25:refnum<visa-resource-name>)  [unwired: 1 in, 2 out]
      n34 = property class="Clust (strict)"(reference=w77) -> ("Value"=w28:T41)  [unwired: 1 in, 2 out]
      n35 = property class="Str"(reference=w78) -> ("Value"=w85:string)  [unwired: 1 in, 2 out]
      n36 = property class="DigNum (strict)"(reference=w83) -> ("Value"=w86:u16)  [unwired: 1 in, 2 out]
      n37 = property class="DigNum (strict)"(reference=w37) -> ("Value"=w36:dbl)  [unwired: 1 in, 2 out]
      n38 = property class="DAQmxName"(reference=w82) -> ("Value"=w87:string)  [unwired: 1 in, 2 out]
      n39 = property class="DAQmxName"(reference=w81) -> ("Value"=w88:string)  [unwired: 1 in, 2 out]
      n40 = property class="DAQmxName"(reference=w80) -> ("Value"=w89:string)  [unwired: 1 in, 2 out]
      n41 = property class="DAQmxName"(reference=w39) -> ("Value"=w38:string)  [unwired: 1 in, 2 out]
      n42 = property class="DAQmxName"(reference=w79) -> ("Value"=w90:string)  [unwired: 1 in, 2 out]
      n43 = property class="DAQmxName"(reference=w84) -> ("Value"=w40:string)  [unwired: 1 in, 2 out]
      n44 = property class="Bool (strict)"(reference=w73) -> ("Value"=w71:bool)  [unwired: 1 in, 2 out]
      n45 = property class="Bool (strict)"(reference=w72) -> ("Value"=w70:bool)  [unwired: 1 in, 2 out]
      n46 = property class="Str"(reference=w69) -> ("Value"=w68:string)  [unwired: 1 in, 2 out]
      n47 = property class="Bool (strict)"(reference=w67) -> ("Value"=w66:bool)  [unwired: 1 in, 2 out]
      n48 = property class="Bool (strict)"(reference=w65) -> ("Value"=w64:bool)  [unwired: 1 in, 2 out]
      n49 = property class="Bool (strict)"(reference=w59) -> ("Value"=w58:bool)  [unwired: 1 in, 2 out]
      n50 = property class="Arr (strict)"(reference=w63) -> ("Value"=w62:T2)  [unwired: 1 in, 2 out]
      n51 = property class="Clust (strict)"(reference=w61) -> ("Value"=w60:T42)  [unwired: 1 in, 2 out]
      n52 = property class="DigNum (strict)"(reference=w54) -> ("Value"=w52:u8)  [unwired: 1 in, 2 out]
      n53 = property class="DigNum (strict)"(reference=w55) -> ("Value"=w53:dbl)  [unwired: 1 in, 2 out]
      n54 = property class="Enum (strict)"(reference=w35) -> ("Value"=w34:enum16{"Full functionality", "Demo mode"})  [unwired: 1 in, 2 out]
      n55 = Not Equal To 0?(x=w34) -> (x != 0?=w33:bool)
      n56 = Bundle By Name(cluster=T7 {"Pockels cal.Zoom"=0, "Pockels cal.Dwell time (µs)"=0.0} ("Calibration settings"), "Pockels cal.Zoom"=w52, "Pockels cal.Dwell time (µs)"=w53) -> (w51:T7)
      n57 = In Range and Coerce(upper limit=u16 100, x=w46, lower limit=u16 0) -> (coerced(x)=w45:u16)  [unwired: 1 out]
      n58 = global write "General Globals.vi" "DevPC - No hardware"(w33) -> ()
      n59 = To Long Integer(number=w45) -> (32bit integer=w44:i32)
      n60 = disable-structure shown="Enabled" {
        disable-tunnel: w28 -> [w91 w99]
        disable-tunnel: [w93 w98] -> w26
        disable-tunnel: [w92 w97] -> w23
        disable-tunnel: w24 -> [_ w96]
        disable-tunnel: [_ w95] -> w22
        disable-tunnel: [_ w94] -> w21
        frame Disabled {
          n61 = call "Sys config-Maintain hidden config values.vi"("Existing System Configuration"=w91) -> (2:w92, "Updated System Configuration"=w93:T43)  [unwired: 9 in]
        }
        frame Enabled {
          n62 = call "Split Control FPGA cluster.vi"("New DAQ FPGA Configuration"=w96, "New Control FPGA Configuration"=w99) -> ("DAQ FPGA System Config"=w94:T22, "Control FPGA System Config"=w95:T23, "DAQ FPGA HW Config"=w97:T33, "Control FPGA HW Config"=w98:T18)  [unwired: 5 in, 1 out]
        }
      }
      n63 = Index Array(array=w49, index=w44) -> (element=w42:string)
      n64 = Decimal String To Number(string=w42) -> (number=w41:i32)  [unwired: 2 in, 1 out]
      n65 = To Double Precision Float(number=w41) -> (double precision float=w20:dbl)
      n66 = Bundle By Name(cluster=w57, "Control Sys. HW config"=w22, "DAQ FPGA HW Config"=w21, "XY Stage.COM port"=w25, "Encoder.IP address"=w85, "Encoder.Port"=w86, "Encoder.Wheel radius (cm)"=w36, "DAQmx Chan.Pockels AO"=w87, "DAQmx Chan.Hard shutter AO"=w88, "DAQmx Chan.PMT AOs"=w89, "DAQmx Chan.Power meter AI"=w38, "Cam VidRec.DO flag-Video record"=w90, "Cam VidRec.DO flag-Trial start"=w40, "XY stage available"=w71, "Encoder available"=w70, "Computer MAC address"=w68, "Externalise Triggers"=w66, "VidRec available"=w64, "MC Supported"=w58) -> (w74:T31)
      n67 = Bundle By Name(cluster=w29, "Control system"=w26, "DAQ FPGA System"=w23, "Laser wavelength (nm)"=w20) -> (w27:T21)
    }
    frame "Set" {
      n68 = call "Create Control FPGA cluster.vi"("System Config"=w100, "Hardware Configuration"=w102) -> ("output cluster"=w101:T43)  [unwired: 9 in]
      n69 = call "Create DAQ FPGA cluster.vi"("System Config"=w100, "Hardware Configuration"=w102) -> ("DAQ FPGA config cluster"=w103:T40)  [unwired: 9 in]
      n70 = Unbundle By Name(w102) -> ("Cam VidRec.DO flag-Video record"=w143:tag)
      n71 = global read "General Globals.vi" "DevPC - No hardware"() -> (w109:bool)
      n72 = Unbundle By Name(w102) -> ("DAQmx Chan.Hard shutter AO"=w146:tag)
      n73 = Unbundle By Name(w102) -> ("Cam VidRec.DO flag-Trial start"=w144:tag)
      n74 = Unbundle By Name(w102) -> ("DAQmx Chan.Power meter AI"=w114:tag)
      n75 = Unbundle By Name(w100) -> ("Laser wavelength (nm)"=w116:dbl)
      n76 = Unbundle By Name(w102) -> ("Encoder.Wheel radius (cm)"=w112:dbl)
      n77 = global read "gl_Calibration globals.vi" "Pockels cal.Dwell time (µs)"() -> (w118:dbl)
      n78 = Unbundle By Name(w102) -> ("DAQmx Chan.Pockels AO"=w147:tag)
      n79 = Unbundle By Name(w105) -> ("Pockels cal.Dwell time (µs)"=w122:refnum<vi>)
      n80 = Unbundle By Name(w105) -> ("DAQ FPGA config cluster"=w158:refnum<vi>)
      n81 = Unbundle By Name(w102) -> ("DAQmx Chan.PMT AOs"=w145:tag)
      n82 = Unbundle By Name(w105) -> ("Computer MAC address"=w138:refnum<vi>)
      n83 = Unbundle By Name(w102) -> ("Computer MAC address"=w137:string)
      n84 = Unbundle By Name(w105) -> ("General trigger settings"=w106:refnum<vi>)
      n85 = Unbundle By Name(w105) -> ("MC Supported"=w127:refnum<vi>)
      n86 = Unbundle By Name(w102) -> ("XY stage available"=w142:bool)
      n87 = Unbundle By Name(w102) -> ("VidRec available"=w133:bool)
      n88 = Unbundle By Name(w102) -> ("Encoder available"=w139:bool)
      n89 = Unbundle By Name(w105) -> ("Triggers output setup"=w132:refnum<vi>)
      n90 = Unbundle By Name(w105) -> ("Cam VidRec available"=w134:refnum<vi>)
      n91 = Unbundle By Name(w105) -> ("DO flag-Video record"=w156:refnum<vi>)
      n92 = Unbundle By Name(w102) -> ("XY Stage.COM port"=w150:refnum<visa-resource-name>)
      n93 = Unbundle By Name(w105) -> ("XY stage COM port"=w159:refnum<vi>)
      n94 = Unbundle By Name(w105) -> ("Encoder IP address"=w157:refnum<vi>)
      n95 = Unbundle By Name(w102) -> ("Encoder.IP address"=w149:string)
      n96 = Unbundle By Name(w105) -> ("Externalise Triggers"=w135:refnum<vi>)
      n97 = Unbundle By Name(w102) -> ("Externalise Triggers"=w136:bool)
      n98 = Unbundle By Name(w105) -> ("Wheel radius (cm)"=w111:refnum<vi>)
      n99 = Unbundle By Name(w105) -> ("XY stage available"=w141:refnum<vi>)
      n100 = Unbundle By Name(w105) -> ("Encoder available"=w140:refnum<vi>)
      n101 = Unbundle By Name(w105) -> ("DO flag-Trial start"=w151:refnum<vi>)
      n102 = global read "gl_Calibration globals.vi" "Pockels cal.Zoom"() -> (w119:u8)
      n103 = Unbundle By Name(w105) -> ("AOL Properties"=w128:refnum<vi>)
      n104 = Unbundle By Name(w105) -> ("Pockels cal.Zoom"=w121:refnum<vi>)
      n105 = Unbundle By Name(w102) -> ("MC Supported"=w126:bool)
      n106 = Unbundle By Name(w105) -> ("Hard shutter AO"=w154:refnum<vi>)
      n107 = Unbundle By Name(w105) -> ("Power meter AI"=w113:refnum<vi>)
      n108 = Unbundle By Name(w105) -> ("Control system"=w124:T44)
      n109 = Unbundle By Name(w105) -> ("Encoder port"=w152:refnum<vi>)
      n110 = Unbundle By Name(w102) -> ("Encoder.Port"=w148:u16)
      n111 = Unbundle By Name(w105) -> ("Demo mode"=w110:refnum<vi>)
      n112 = Unbundle By Name(w105) -> ("Pockels AO"=w153:refnum<vi>)
      n113 = Unbundle By Name(w105) -> ("PMT AOs"=w155:refnum<vi>)
      n114 = Boolean To (0,1)(Boolean=w109) -> (0, 1=w108:i16)
      n115 = call "fgv_Triggers Output Setup.vi"("Function"=HW_config_states_enum."Read all") -> ("General trigger settings"=w104:T4, "Triggers output setup"=w125:T2)  [unwired: 8 in, 1 out]
      n116 = call "fgv_AOL Properties.vi"("Function"=HW_config_states_enum."Read all") -> ("AOL Properties out"=w129:T6)  [unwired: 9 in, 1 out]
      n117 = To Unsigned Word Integer(number=w116) -> (unsigned 16bit integer=w115:u16)
      n118 = To Unsigned Word Integer(number=w108) -> (unsigned 16bit integer=w107:u16)
      n119 = property class="VISAName"(reference=w159, "Value"=w150) -> ()  [unwired: 1 in, 2 out]
      n120 = property class="Bool (strict)"(reference=w140, "Value"=w139) -> ()  [unwired: 1 in, 2 out]
      n121 = property class="Str"(reference=w157, "Value"=w149) -> ()  [unwired: 1 in, 2 out]
      n122 = property class="DigNum (strict)"(reference=w152, "Value"=w148) -> ()  [unwired: 1 in, 2 out]
      n123 = property class="DigNum (strict)"(reference=w111, "Value"=w112) -> ()  [unwired: 1 in, 2 out]
      n124 = property class="DAQmxName"(reference=w153, "Value"=w147) -> ()  [unwired: 1 in, 2 out]
      n125 = property class="DAQmxName"(reference=w154, "Value"=w146) -> ()  [unwired: 1 in, 2 out]
      n126 = property class="DAQmxName"(reference=w155, "Value"=w145) -> ()  [unwired: 1 in, 2 out]
      n127 = property class="DAQmxName"(reference=w113, "Value"=w114) -> ()  [unwired: 1 in, 2 out]
      n128 = property class="Bool (strict)"(reference=w141, "Value"=w142) -> ()  [unwired: 1 in, 2 out]
      n129 = property class="Str"(reference=w138, "Value"=w137) -> ()  [unwired: 1 in, 2 out]
      n130 = property class="Bool (strict)"(reference=w135, "Value"=w136) -> ()  [unwired: 1 in, 2 out]
      n131 = property class="Bool (strict)"(reference=w134, "Value"=w133) -> ()  [unwired: 1 in, 2 out]
      n132 = property class="DAQmxName"(reference=w156, "Value"=w143) -> ()  [unwired: 1 in, 2 out]
      n133 = property class="DAQmxName"(reference=w151, "Value"=w144) -> ()  [unwired: 1 in, 2 out]
      n134 = property class="Arr (strict)"(reference=w132, "Value"=w125) -> ()  [unwired: 1 in, 2 out]
      n135 = property class="Clust (strict)"(reference=w106, "Value"=w104) -> ()  [unwired: 1 in, 2 out]
      n136 = property class="Clust (strict)"(reference=w128, "Value"=w129) -> ()  [unwired: 1 in, 2 out]
      n137 = property class="Bool (strict)"(reference=w127, "Value"=w126) -> ()  [unwired: 1 in, 2 out]
      n138 = property class="DigNum (strict)"(reference=w121, "Value"=w119) -> ()  [unwired: 1 in, 2 out]
      n139 = property class="DigNum (strict)"(reference=w122, "Value"=w118) -> ()  [unwired: 1 in, 2 out]
      n140 = call "Sys config window-Set wavelengths ring.vi"("Laser wavelength (nm)"=w115, "System Config window refs"=w105) -> ()  [unwired: 9 in, 1 out]
      n141 = property class="Enum (strict)"(reference=w110, "Value"=w107) -> ()  [unwired: 1 in, 2 out]
      n142 = property class="Clust (strict)"(reference=w124, "Value"=w101) -> ()  [unwired: 1 in, 2 out]
      n143 = property class="Clust (strict)"(reference=w158, "Value"=w103) -> ()  [unwired: 1 in, 2 out]
      n144 = Bundle By Name(cluster=T7 {"Pockels cal.Zoom"=0, "Pockels cal.Dwell time (µs)"=0.0} ("Calibration settings"), "Pockels cal.Zoom"=w119, "Pockels cal.Dwell time (µs)"=w118) -> (w117:T7)
    }
  }
  "error out" <- w17
  n145 = Bundle By Name(cluster=T30 {"Triggers output setup"=[], "General trigger settings"={"Trigger 1 function"=enum."Encoder trigger", "Triggers loop clock (MHz)"=80.0}, "Calibration settings"={"Pockels cal.Zoom"=0, "Pockels cal.Dwell time (µs)"=0.0}, "Hardware Configuration"={"Dev. PC"=FALSE, "Swap XY on stage"=FALSE, "No of AOD"=0, "MC Supported"=FALSE, "Axial MC"=FALSE, "Computer MAC address"="", "Externalise Triggers"=FALSE, "Trigger HW config"={"Available Device List"=0, "Device Address"=""}, "DAQmx Chan"={"Pockels AO"="", "Hard shutter AO"="", "PMT AOs"="", "Galvo AOs"="", "Power meter AI"=""}, "XY stage available"=FALSE, "XY Stage"={"COM port"="", "Baudrate"=0, "Type"=""}, "Z stage available"=FALSE, "Z Stage config cluster"={"COM port"="COM7", "Baudrate"=0, "Type"=""}, "Encoder available"=FALSE, "Encoder"={"IP address"="224.0.1.103", "Port"=7000, "Wheel radius (cm)"=16.0, "Encoder Trigger"=""}, "VidRec available"=FALSE, "Cam VidRec"={"DO flag-Video record"="", "DO flag-Trial start"=""}, "Laser Power Control HW config"={"Laser Power Control"="", "Laser Power Modulation Control"=enum."FPGA"}, "Laser 1 available"=FALSE, "Laser 1 config cluster"={"COM port"="COM7", "Baud Rate"=0, "Type"=""}, "Prechirper 1 available"=FALSE, "Prechirper 1 config cluster"={"Type"="", "Baud Rate"=0, "COM port"="COM7"}, "Control system.FPGA available?"=FALSE, "Control Sys. HW config"={"Control system.FPGA Type"=enum."Virtex 7", "Control system.Network adapter name"="", "Control system.MAC address"="", "Control system.Ethernet Port"=0, "Control system.Ethernet Port Opened"=FALSE}, "DAQ FPGA HW Config"={"FGPA Ref"=refnum, "Target"="RIO0", "input card type"=enum."AC Card"}, "PMT Voltage Range"={"PMT Voltage Lower Limit"=110.0, "PMT Voltage Upper Limit"=135.0}}, "System Config"={"Laser wavelength (nm)"=920.0, "DAQ FPGA System"={"Clock Freq (MHz) "=200.0, "Samples Wait after Trigger"=5080, "AOD fill"=4900, "StartupDelay"=0, "Slip Cycle (clock cycles)"=600000, "Add Cycle"=TRUE}, "Control system"={"AOD 1 Amplitude"=0, "AOD 2 Amplitude"=0, "AOD 3 Amplitude"=0, "AOD 4 Amplitude"=0, "AOD 5 Amplitude"=0, "AOD 6 Amplitude"=0, "T0 (ns)"=0.0, "Ta (ns)"=0.0, "Data Time Interval (ns)"=0.0, "Ctrl FPGA Clock (MHz)"=240.0}}, "Calibration config."={"Current Objective"="", "Objective Settings"=[], "PreChirper Values Preset ?"=FALSE, "PreChirper Settings"=[], "PreChirper Constants"={"a 1"=0, "b 1"=0, "c 1"=0, "a 2"=0, "b 2"=0, "c 2"=0, "lmin"=0, "lmax"=0}}, "General Setup"={"Microscope ID"="003", "Microscope Type"="AOLM", "Revision Number"="1.0.0.0", "Advanced Imaging"=FALSE, "Error Logging"=FALSE, "Performance Monitoring"=FALSE, "Max Allowed Trial Length"=15.0, "Initial Scan Resolution"=15.0, "Initial Acceptance Angle"=15.0, "Initial Laser Wavelength"=15.0, "Initial Dwell Time"=15.0}, "AOD Settings - distilled"={"AOD 1 thickness (mm)"=135.0, "AOD 2 thickness (mm)"=135.0, "AOD 3 thickness (mm)"=15.0, "AOD 4 thickness (mm)"=50.0, "AOD 1-2 separation (mm)"=50.0, "AOD 2-3 separation (mm)"=50.0, "AOD 3-4 separation (mm)"=15.0, "AOD 1 Centre (mm)"=1.0, "AOD 2 Centre (mm)"=1.0, "AOD 3 Centre (mm)"=1.0, "AOD 4 Centre (mm)"=1.0, "AOD 1 X Offset"=1.0, "AOD 2 X Offset"=1.0, "AOD 3 X Offset"=1.0, "AOD 4 X Offset"=1.0, "AOD 1 Y Offset"=0.0, "AOD 2 Y Offset"=1.0, "AOD 3 Y Offset"=1.0, "AOD 4 Y Offset"=2.22, "Timing Offset AOD 1"=0.0, "Timing Offset AOD 2"=0.0, "Timing Offset AOD 3"=0.0, "Timing Offset AOD 4"=0.0, "AOL centre wavelength (nm)"=0.0, "AOL centre frequency (MHz)"=0.0, "Pair deflection ratio"=0.0, "AOL aperture (mm)"=0.0, "AOD fill time (us)"=1.0, "Diffraction mode"=20000.0, "Crystal length (mm)"=20000.0, "Acoustic velocity (m/s)"=60.0, "AOD Ord. Refractive index"=512.0}} ("Initial configuration"), "System Config"=w6, "Hardware Configuration"=w7, "Triggers output setup"=w16, "General trigger settings"=w11, "AOL Properties"=w12, "Calibration settings"=w13) -> (→"output cluster":T30)
